vi "Open Bundle.vi"(8 "error in (no error)":errorcluster, 11 "Bundle Builder in":refnum<class "Bundle Builder.lvclass">) -> (0 "error out":errorcluster, 1 "Custom Actions File Names":string[](array[string]), 2 "Product List File Names":string[](array[string]), 3 "Bundle Builder out":refnum<class "Bundle Builder.lvclass">, 4 "Bundle Filename":string)   [LabVIEW 2020, in "Bundle Builder.lvclass"]
uses:
  Bundle Builder.lvclass
  Bundle Builder.lvclass/Bundle Builder.ctl
  C:/Users/chihong/Documents/Repos/StsCustomBundleBuilder/Code/StsCustomBundleBuilderLib/StsCustomBundleBuilderLib/bin/Debug/StsCustomBundleBuilderLib.dll
  StsCustomBundleBuilderLib/StsCustomBundleBuilderLib/bin/Debug/StsCustomBundleBuilderLib.dll
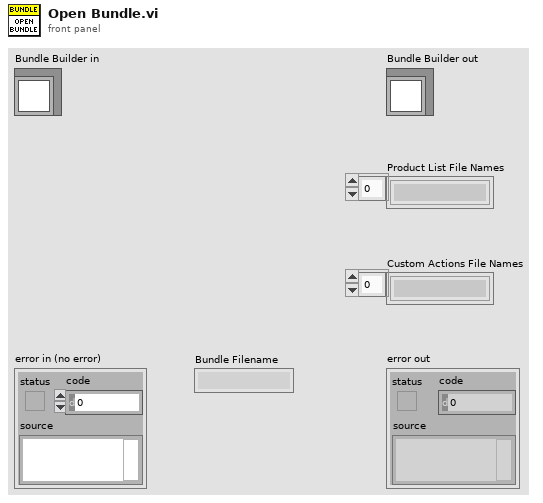
[diagram p1: front panel]
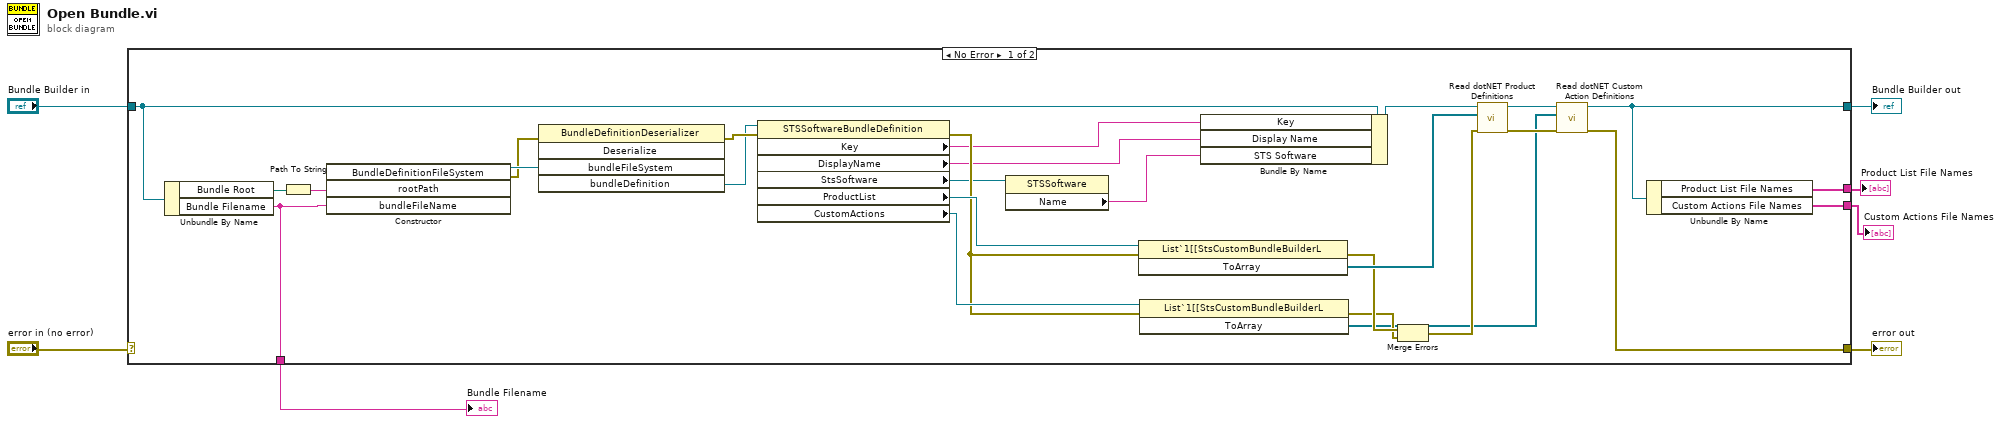
[diagram p0: block diagram]
diagram:
  n1 = case shown="No Error" "error in (no error)" {
    selector: "error in (no error)" -> [_ w36]
    tunnel: [w17 w36] -> w6
    tunnel: [w16 w35] -> w4
    tunnel: "Bundle Builder in" -> [w34 w35]
    tunnel: [w25 _] -> w3
    tunnel: [w15 _] -> w2
    tunnel: [w14 _] -> w1
    frame No Error {
      n2 = Unbundle By Name(w34) -> ("Bundle Root"=w33:path, "Bundle Filename"=w25:string)
      n3 = Path To String(path=w33) -> (string=w32:string)
      n4 = constructor class="BundleDefinitionFileSystem"("rootPath"=w32, "bundleFileName"=w25) -> (reference out=w31:refnum<k24>, error out=w30:errorcluster)  [unwired: 3 in, 3 out]
      n5 = invoke class="BundleDefinitionDeserializer" method="Deserialize"(error in=w30, "bundleFileSystem"=w31) -> (error out=w26:errorcluster, "bundleDefinition"=w13:refnum<k24>)  [unwired: 3 in, 3 out]
      n6 = property class="STSSoftwareBundleDefinition"(reference=w13, error in=w26) -> (error out=w27:errorcluster, "Key"=w8:string, "DisplayName"=w9:string, "StsSoftware"=w11:refnum<k24>, "ProductList"=w29:refnum<k24>, "CustomActions"=w28:refnum<k24>)  [unwired: 1 out]
      n7 = property class="STSSoftware"(reference=w11) -> ("Name"=w10:string)  [unwired: 1 in, 2 out]
      n8 = invoke class="List`1[[StsCustomBundleBuilderL" method="ToArray"(reference=w29, error in=w27) -> (error out=w22:errorcluster, "ToArray"=w23:refnum<k24>[])  [unwired: 1 in, 1 out]
      n9 = invoke class="List`1[[StsCustomBundleBuilderL" method="ToArray"(reference=w28, error in=w27) -> (error out=w19:errorcluster, "ToArray"=w18:refnum<k24>[])  [unwired: 1 in, 1 out]
      n10 = Bundle By Name(cluster=w34, "Key"=w8, "Display Name"=w9, "STS Software"=w10) -> (w12:refnum<class "Bundle Builder.lvclass">)
      n11 = Merge Errors(w22, w19) -> (w20:errorcluster)
      n12 = call "Read dotNET Product Definitions.vi"("error in (no error)"=w20, "Product Definitions"=w23, "Bundle Builder in"=w12) -> ("error out"=w21:errorcluster, "Bundle Builder out"=w24:refnum<class "Bundle Builder.lvclass">)  [unwired: 7 in]
      n13 = call "Read dotNET Custom Action Definitions.vi"("error in (no error)"=w21, "Custom Action Definitions"=w18, "Bundle Builder in"=w24) -> ("error out"=w17:errorcluster, "Bundle Builder out"=w16:refnum<class "Bundle Builder.lvclass">)  [unwired: 7 in]
      n14 = Unbundle By Name(w16) -> ("Product List File Names"=w15:string[], "Custom Actions File Names"=w14:string[])
    }
    frame Error {
    }
  }
  "error out" <- w6
  "Bundle Builder out" <- w4
  "Product List File Names" <- w2
  "Custom Actions File Names" <- w1
  "Bundle Filename" <- w3
